vi "Run Panel VI.vi"(8 "error in (no error)":errorcluster, 11 "Panel in":refnum<class "Panel.lvclass">) -> (0 "error out":errorcluster, 3 "Panel out":refnum<class "Panel.lvclass">)   [LabVIEW 2018, in "OOPanel.lvlib" / "Panel.lvclass"]
uses:
  Panel.lvclass
  Visibility State.ctl
  <vilib>/ErrorRing/Error Ring.xnode
  <vilib>/Utility/error.llb/Error Cluster From Error Code.vi
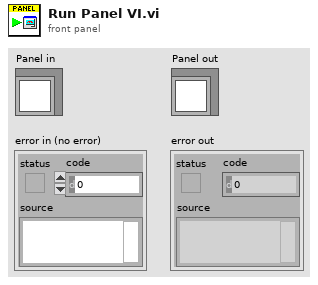
[diagram p1: front panel]
types:
  T1 = typedef "OOPanel.lvlib/Panel.lvclass/Visibility State.ctl" = enum16{"Idle", "Closed", "Hidden", "Visible", "Subpanel"}
  T2 = typedef "OOPanel.lvlib/Panel.lvclass/Ref Data.ctl" = cluster{"Panel Ref":refnum<vi>, "SubPanel":refnum<vi>, "Close":bool, "Running":bool, "State":T1}
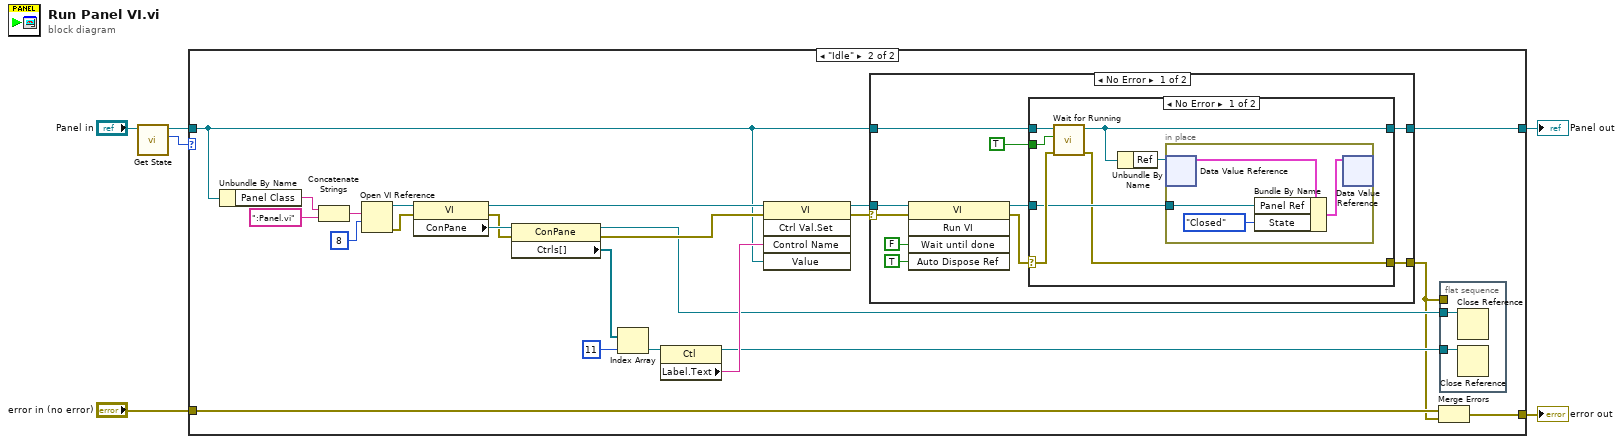
[diagram p0: block diagram]
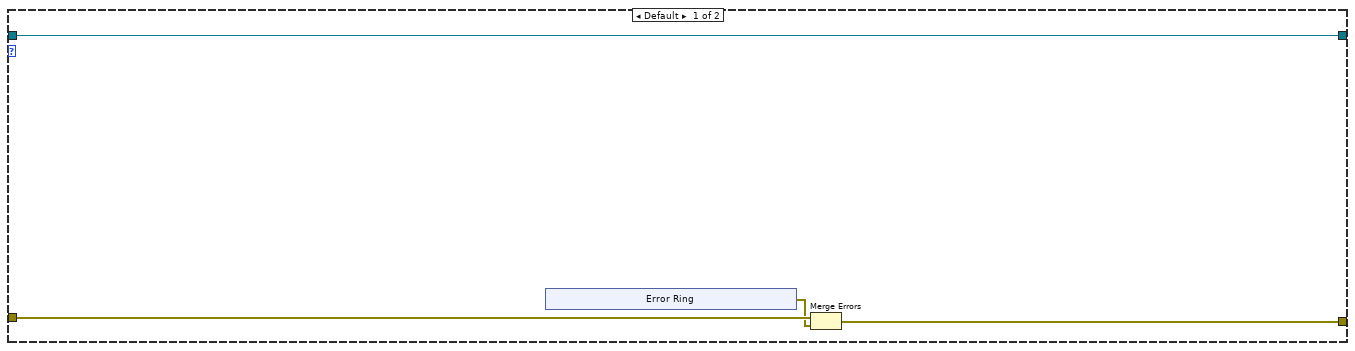
[diagram p2: hidden frame]
diagram:
  n1 = call "Get State.vi"("Panel in"="Panel in") -> ("State"=w1:T1, "Panel out"=w2:refnum<class "Panel.lvclass">)  [unwired: 8 in, 1 out]
  n2 = case shown="\"Idle\"" w1 {
    tunnel: "error in (no error)" -> [w9 w37]
    tunnel: [w10 w21] -> w5
    tunnel: [w7 w20] -> w4
    tunnel: w2 -> [w10 w16]
    frame Default {
      n3 = xnode "Error Ring"() -> ("error out"=w8:errorcluster)
      n4 = Merge Errors(w9, w8) -> (w7:errorcluster)
    }
    frame "Idle" {
      n5 = Unbundle By Name(w16) -> ("Panel Class"=w15:string)
      n6 = Concatenate Strings(w15, ":Panel.vi" ("string")) -> (w35:string)
      n7 = Open VI Reference(vi path=w35, options=8) -> (vi reference=w34:refnum<vi>, error out=w33:errorcluster)  [unwired: 4 in]
      n8 = property class="VI"(reference=w34, error in=w33) -> (reference out=w29:refnum<vi>, error out=w27:errorcluster, "ConPane"=w32:refnum<vi>)
      n9 = property class="ConPane"(reference=w32, error in=w27) -> (reference out=w22:refnum<vi>, error out=w26:errorcluster, "Ctrls[]"=w31:refnum<vi>[])
      n10 = Index Array(array=w31, index=11) -> (element=w30:refnum<vi>)
      n11 = property class="Ctl"(reference=w30) -> (reference out=w23:refnum<vi>, "Label.Text"=w28:string)  [unwired: 1 in, 1 out]
      n12 = invoke class="VI" method="Ctrl Val.Set"(reference=w29, error in=w26, "Control Name"=w28, "Value"=w16) -> (reference out=w18:refnum<vi>, error out=w24:errorcluster)  [unwired: 1 in, 3 out]
      n13 = case shown="No Error" w24 {
        selector: w24 -> [w46 w63]
        tunnel: w18 -> [w47 _]
        tunnel: [w40 w63] -> w19
        tunnel: w16 -> [w44 w64]
        tunnel: [w43 w64] -> w21
        frame No Error {
          n14 = invoke class="VI" method="Run VI"(reference=w47, error in=w46, "Wait until done"=FALSE ("Wait Until Done"), "Auto Dispose Ref"=TRUE ("Auto Dispose Reference")) -> (reference out=w45:refnum<vi>, error out=w41:errorcluster)  [unwired: 1 in, 3 out]
          n15 = case shown="No Error" w41 {
            selector: w41 -> [w52 w62]
            tunnel: w45 -> [w51 _]
            tunnel: w44 -> [w55 w61]
            tunnel: [w54 w61] -> w43
            tunnel: TRUE ("Running") -> [w53 _]
            tunnel: [w50 w62] -> w40
            frame No Error {
              n16 = call "Wait for Running.vi"("error in (no error)"=w52, "Running"=w53, "Panel in"=w55) -> ("error out"=w50:errorcluster, "Panel out"=w54:refnum<class "Panel.lvclass">)  [unwired: 7 in]
              n17 = Unbundle By Name(w54) -> ("Ref"=w56:refnum<data-value>)
              n18 = in-place {
                in-place-border: w51 -> [w57]
                n19 = in-place-dvr #1(w56) -> (w60:T2)  [unwired: 1 out]
                n20 = Bundle By Name(cluster=w60, "Panel Ref"=w57, "State"=Visibility_State."Closed") -> (w59:T2)
                n21 = in-place-dvr #1(w59) -> ()  [unwired: 2 out]
              }
            }
            frame Error {
            }
          }
        }
        frame Error {
        }
      }
      n22 = Merge Errors(w37, w19) -> (w20:errorcluster)
      n23 = flat-sequence {
        tunnel: w23 -> [w39]
        tunnel: [w38] -> _
        tunnel: w22 -> [w38]
        tunnel: w19 -> [_]
        frame #0 {
          n24 = Close Reference(reference=w38) -> ()  [unwired: 1 in, 1 out]
          n25 = Close Reference(reference=w39) -> ()  [unwired: 1 in, 1 out]
        }
      }
    }
  }
  "error out" <- w4
  "Panel out" <- w5
